vi "Get Default Settings.vi"(8 "error in (no error)":errorcluster, 11 "For Load (F)":bool) -> (0 "error out":errorcluster, 3 "Settings out":T1={"Plug-in Version"="", "Step Values"=[], "Only Execute When Test Running"=TRUE, "Reset Sequence When Test Starts"=TRUE, "Number of Sequence Steps"=0, "Num of Analog Channels"=0, "Num of Digital Channels"=0, "Delay Before Starting Sequence"=0.0, "Default Analog Values"=[], "Default Digital Values"=[], "Max Iterations"=0, "Use last value when stopped"=FALSE, "Prioritize exact values"=FALSE, "Enable advanced step timing"=FALSE, "Enable step conditions"=FALSE, "Show confirmation dialogs"=FALSE, "Start condition"="", "Enable re-triggering"=FALSE, "Stop condition"=""})   [LabVIEW 2024, in "Output Sequencer.lvlib" / "Output Sequencer.lvclass"]
uses:
  Output Sequencer.lvclass
  Settings UI/Types/Settings.ctl
  Settings UI/Types/Step Settings.ctl
  Globals/Global Strings.vi
  Settings UI/Settings UI.lvclass
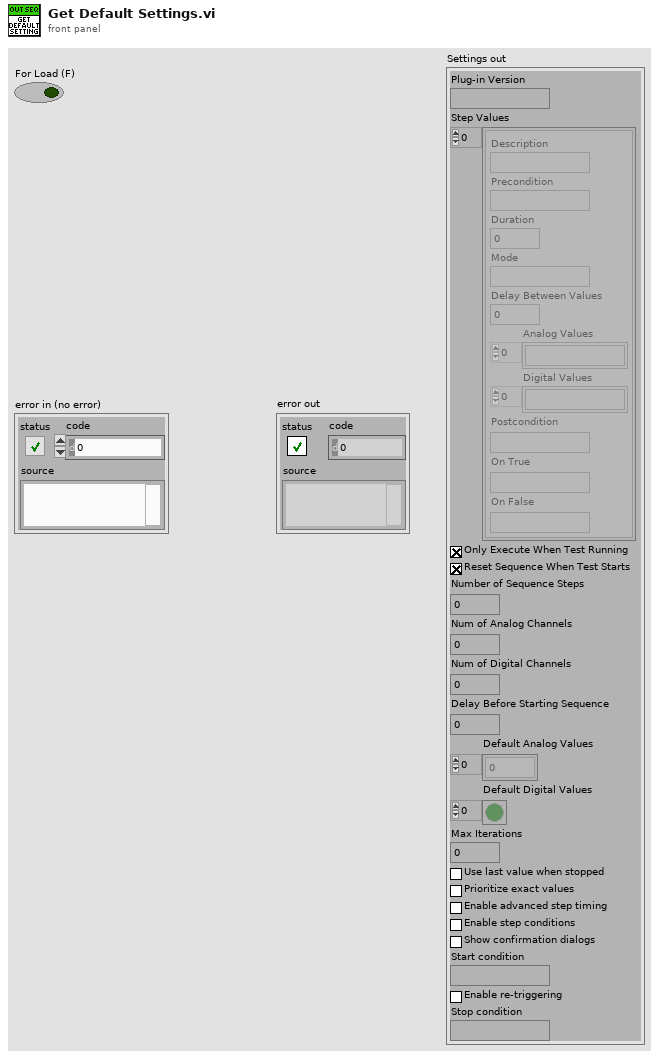
[diagram p1: front panel]
types:
  T1 = typedef "Output Sequencer.lvlib/Settings UI.lvclass/Settings.ctl" = cluster{"Plug-in Version":string, "Step Values":T2[], "Only Execute When Test Running":bool, "Reset Sequence When Test Starts":bool, "Number of Sequence Steps":i32, "Num of Analog Channels":i32, "Num of Digital Channels":i32, "Delay Before Starting Sequence":dbl, "Default Analog Values":dbl[], "Default Digital Values":bool[], "Max Iterations":u32, "Use last value when stopped":bool, "Prioritize exact values":bool, "Enable advanced step timing":bool, "Enable step conditions":bool, "Show confirmation dialogs":bool, "Start condition":string, "Enable re-triggering":bool, "Stop condition":string}
  T2 = typedef "Output Sequencer.lvlib/Settings UI.lvclass/Step Settings.ctl" = cluster{"Description":string, "Precondition":string, "Duration":dbl, "Mode":string, "Delay Between Values":dbl, "Analog Values":string[], "Digital Values":string[], "Postcondition":string, "On True":string, "On False":string}
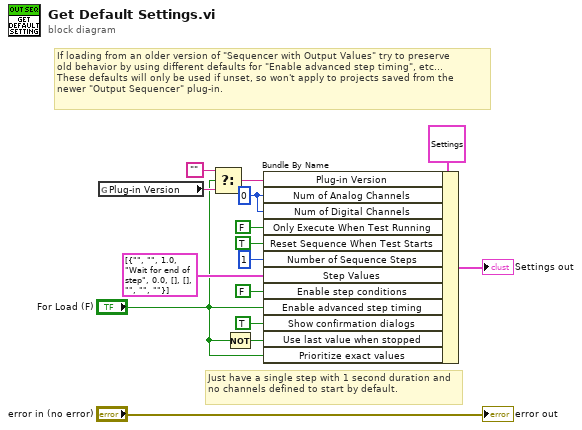
[diagram p0: block diagram]
diagram:
  w14 = 0 ("Num of Analog Channels")
  # "If loading from an older version of \"Sequencer with Output Values\" try to preserve\nold behavior by using different defaults for \"Enable advanced step timing\", etc...\nThese defaults will only be used if unset, so won't apply to projects saved from the\nnewer \"Output Sequencer\" plug-in."
  # "Just have a single step with 1 second duration and no channels defined to start by default."
  n1 = global read "Global Strings.vi" "Plug-in Version"() -> (w5:string)
  n2 = Select(t="", s="For Load (F)", f=w5) -> (s? t:f=w10:string)
  n3 = Not(x="For Load (F)") -> (.not. x?=w3:bool)
  n4 = Bundle By Name(cluster=T1 {"Plug-in Version"="", "Step Values"=[], "Only Execute When Test Running"=FALSE, "Reset Sequence When Test Starts"=FALSE, "Number of Sequence Steps"=0, "Num of Analog Channels"=0, "Num of Digital Channels"=0, "Delay Before Starting Sequence"=0.0, "Default Analog Values"=[], "Default Digital Values"=[], "Max Iterations"=0, "Use last value when stopped"=FALSE, "Prioritize exact values"=FALSE, "Enable advanced step timing"=FALSE, "Enable step conditions"=FALSE, "Show confirmation dialogs"=FALSE, "Start condition"="", "Enable re-triggering"=FALSE, "Stop condition"=""} ("Settings out"), "Plug-in Version"=w10, "Num of Analog Channels"=w14, "Num of Digital Channels"=w14, "Only Execute When Test Running"=FALSE, "Reset Sequence When Test Starts"=TRUE ("Only Execute When Test Running"), "Number of Sequence Steps"=1, "Step Values"=T2[] [{"Description"="", "Precondition"="", "Duration"=1.0, "Mode"="Wait for end of step", "Delay Between Values"=0.0, "Analog Values"=[], "Digital Values"=[], "Postcondition"="", "On True"="", "On False"=""}], "Enable step conditions"=FALSE ("Settings.Enable step conditions"), "Enable advanced step timing"="For Load (F)", "Show confirmation dialogs"=TRUE ("Settings.Enable confirmation dialogs"), "Use last value when stopped"=w3, "Prioritize exact values"="For Load (F)") -> (→"Settings out":T1)
  "error out" <- "error in (no error)"
